vi "CTR_Read.vi"(7 "DeviceIndex":u32, 8 "error in (no error)":errorcluster) -> (0 "error out":errorcluster)   [LabVIEW 2012]
doc: "unsigned long CTR_8254Read(\nunsigned long DeviceIndex - number from 0-31 indicating on which device you wish to read an\n8254 counter\nunsigned long BlockIndex - number indicating which 8254 you wish to read\nunsigned long CounterIndex - number from 0-2 indicating which counter on the specified 8254\nyou wish to read\nunsigned short *pReadValue - a pointer to a WORD in which will be stored the value latched\nand read from the specified counter\n)"
uses:
  Windows/System32/AIOUSB.dll
panel:
  out "pReadValue":u16
  in  "CounterIndex":u32
  in  "BlockIndex":u32
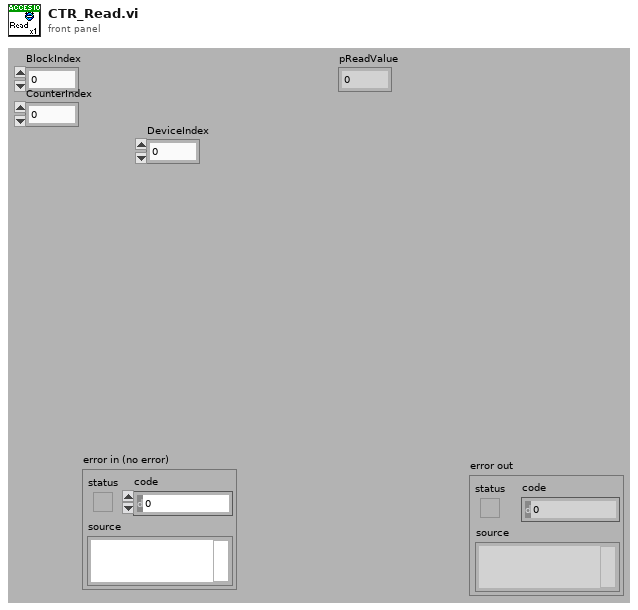
[diagram p1: front panel]
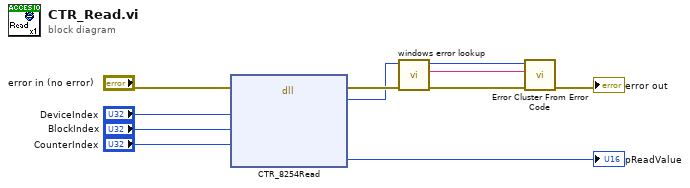
[diagram p0: block diagram]
diagram:
  n1 = dll-call lib="C:/Windows/System32/AIOUSB.dll" fn="CTR_8254Read"(error in="error in (no error)", "DeviceIndex"="DeviceIndex", "BlockIndex"="BlockIndex", "CounterIndex"="CounterIndex") -> (error out=w7:errorcluster, "return type"=w6:u32, "pReadValue"=→"pReadValue":u16)  [unwired: 6 in, 1 out]
  n2 = call "windows error lookup.vi"("error in (no error)"=w7, "Error Code"=w6) -> ("error out"=w9:errorcluster, "error message (\"\")"=w10:string)  [unwired: 8 in]
  n3 = call <vilib>:"Error Cluster From Error Code.vi"("error in (no error)"=w9, "error message (\"\")"=w10, "error code (0)"=w6) -> ("error out"=→"error out":errorcluster)  [unwired: 6 in]
